vi "To Pretty String.vi"(8 "error in (no error)":errorcluster, 11 "JSON Array in":refnum<class "JSON Array.lvclass">) -> (0 "error out":errorcluster, 3 "Pretty Print String":string)   [LabVIEW 2015, in "LVJSON.lvlib" / "JSON Array.lvclass"]
uses:
  JSON Array.lvclass
  JSON Array.lvclass/JSON Array.ctl
  JSON Datatype/JSON Null.lvclass
  LVJSON.lvlib
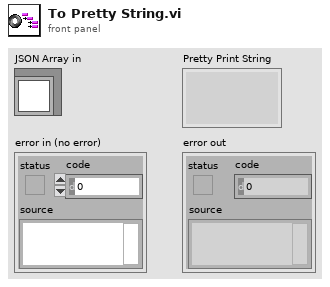
[diagram p1: front panel]
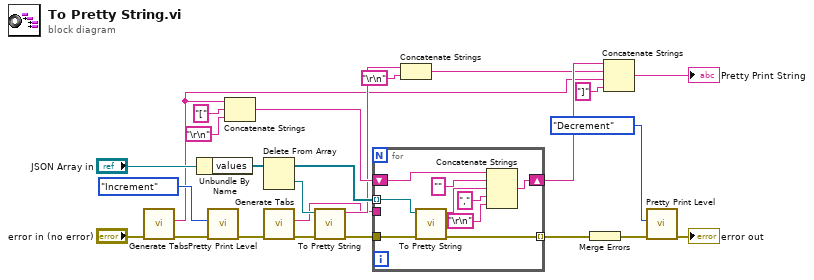
[diagram p0: block diagram]
diagram:
  n1 = call "Generate Tabs.vi"("error in (no error)"="error in (no error)") -> ("error out"=w20:errorcluster, "Tabs"=w4:string)  [unwired: 9 in]
  n2 = Unbundle By Name("JSON Array in") -> ("values"=w1:refnum<class "JSON Null.lvclass">[])
  n3 = call "Pretty Print Level.vi"("error in (no error)"=w20, "Action"=enum16{"Increment", "Decrement", "Get", "Reset"}."Increment") -> ("error out"=w14:errorcluster)  [unwired: 8 in, 1 out]
  n4 = Concatenate Strings(w4, "[" ("string"), "\r\n") -> (w21:string)
  n5 = Delete From Array(array=w1) -> (deleted portion=w12:refnum<class "JSON Null.lvclass">, array with subset deleted=w13:refnum<class "JSON Null.lvclass">[])  [unwired: 2 in]
  n6 = call "Generate Tabs.vi"("error in (no error)"=w14) -> ("error out"=w3:errorcluster, "Tabs"=w5:string)  [unwired: 9 in]
  n7 = call-dynamic "To Pretty String.vi"("error in (no error)"=w3, "JSON Datatype in"=w12) -> ("error out"=w2:errorcluster, "Pretty Print String"=w11:string)  [unwired: 8 in]
  n8 = for {
    tunnel: w13 -> [w34] mode=indexing
    tunnel: w2 -> [w33]
    tunnel: [w32] -> w24 mode=indexing
    shift-right: [w28] -> w9
    shift-left: w21 -> [w27]
    tunnel: w5 -> [_]
    n9 = call-dynamic "To Pretty String.vi"("error in (no error)"=w33, "JSON Datatype in"=w34) -> ("error out"=w32:errorcluster, "Pretty Print String"=w31:string)  [unwired: 8 in]
    n10 = Concatenate Strings(w27, "" ("string"), w31, "," ("string"), "\r\n") -> (w28:string)
  }
  n11 = Concatenate Strings(w11, "\r\n") -> (w8:string)
  n12 = Merge Errors(w24) -> (w18:errorcluster)
  n13 = Concatenate Strings(w9, w8, w4, "]" ("string")) -> (→"Pretty Print String":string)
  n14 = call "Pretty Print Level.vi"("error in (no error)"=w18, "Action"=enum16{"Increment", "Decrement", "Get", "Reset"}."Decrement") -> ("error out"=→"error out":errorcluster)  [unwired: 8 in, 1 out]
